vi "GDX-ACC_PitchAndRoll.vi"() -> ()   [LabVIEW 2019]
uses:
  <vilib>/picture/3D Picture Control/Object/Create Object (drawable).vi
  <vilib>/picture/3D Picture Control/NI_3D Picture Control.lvlib
panel:
  in  "Gyro Percent of Filter":dbl(slide)=75.0 scale=0.0..100.0
  out "Filter":refnum<vi>(3d-picture)
  out "Gyro":refnum<vi>(3d-picture)
  out "Accelerometer":refnum<vi>(3d-picture)
  out "Waveform Chart":cluster{dbl, "Radians Out":dbl, "Filtered":dbl}(graph)
  out "error out":errorcluster
  in  "Stop":bool
  in  "Initialize":bool
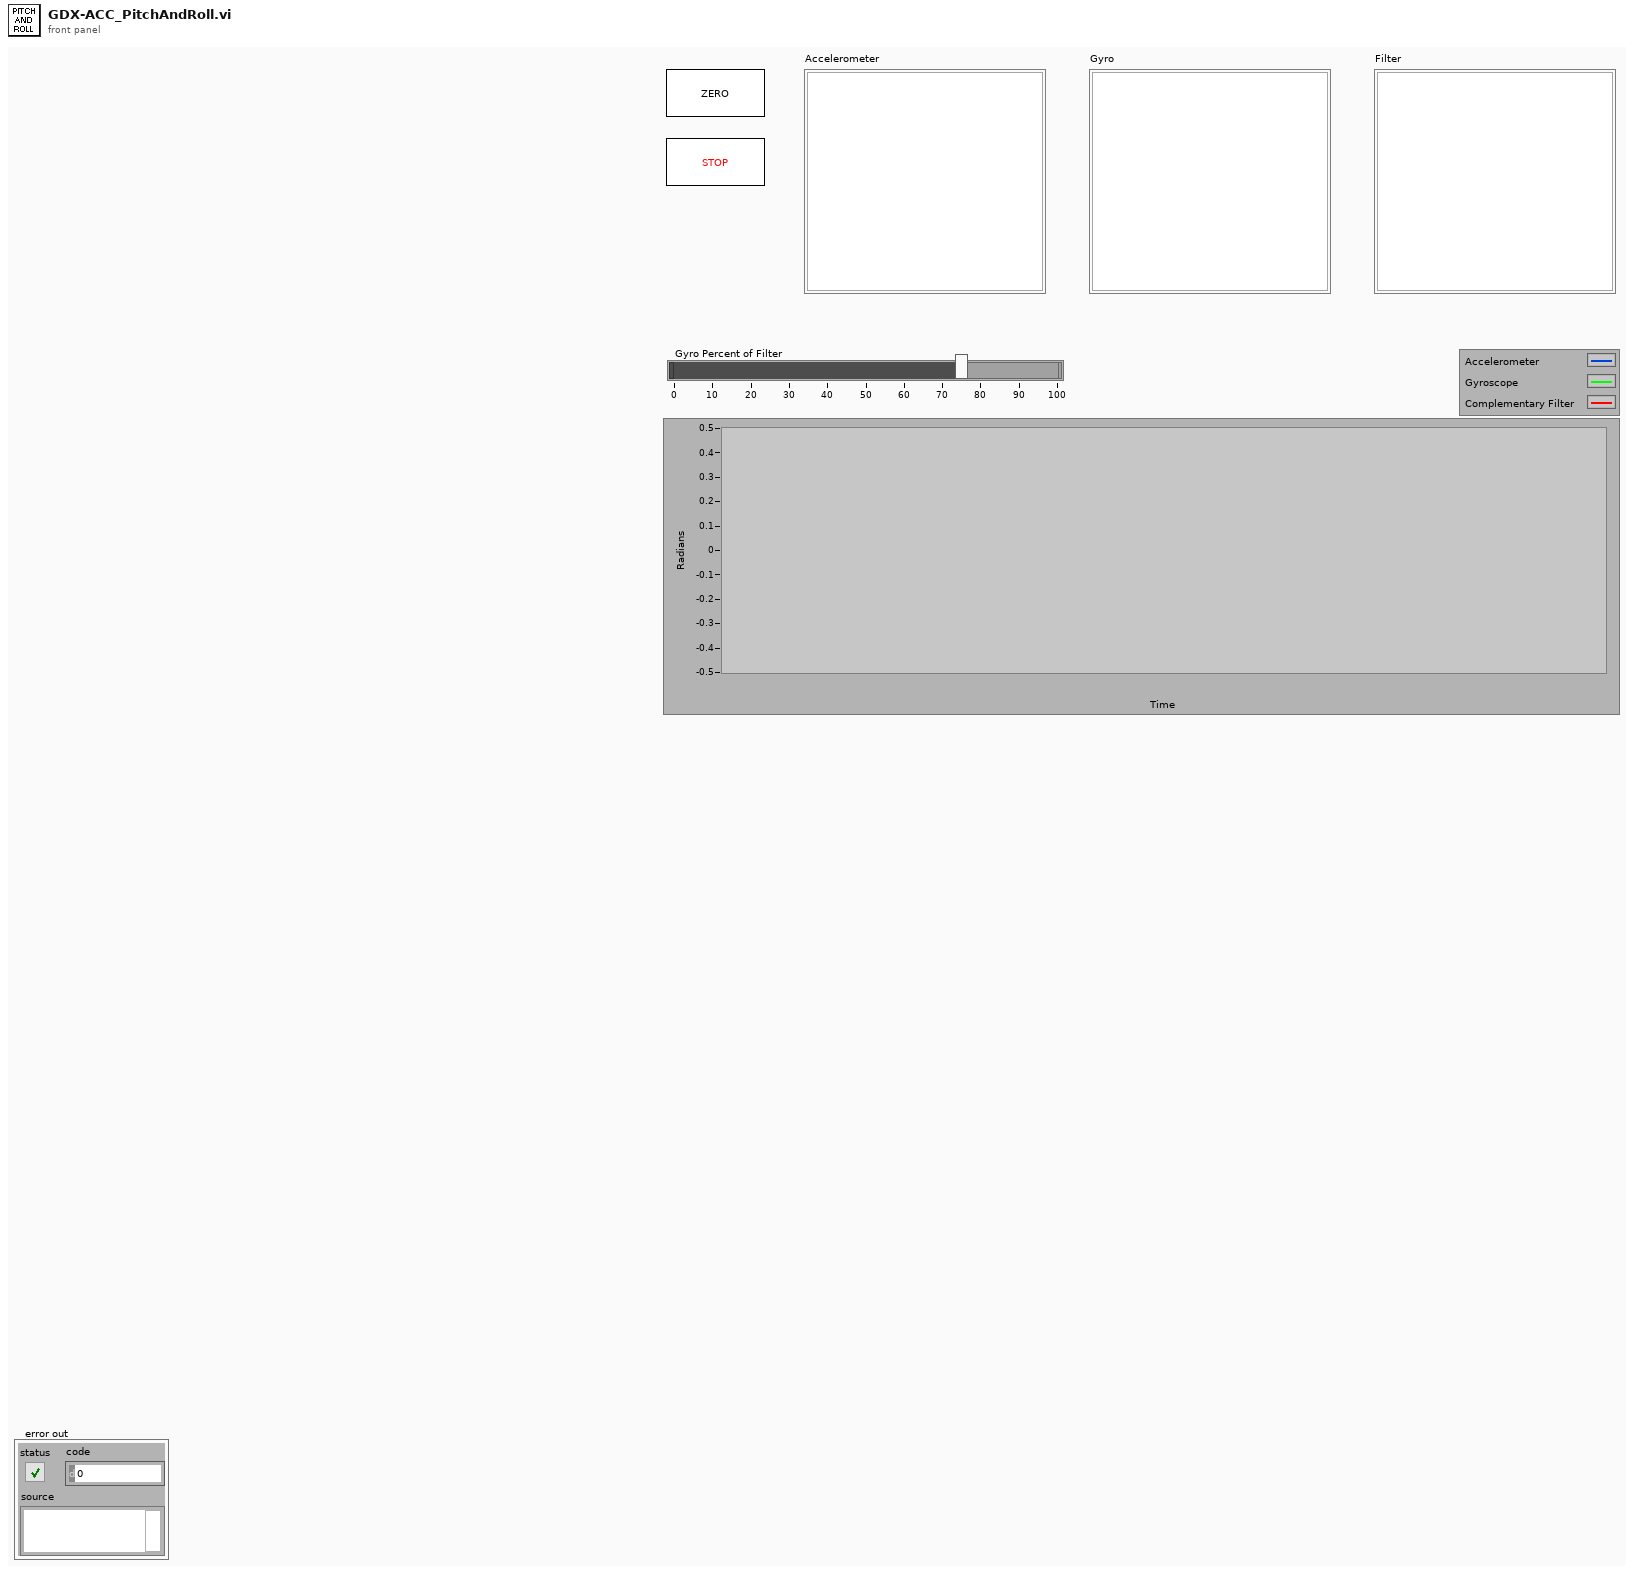
[diagram p1: front panel]
types:
  T1 = enum16{"Activate from Dialog Popup", "Activate All Channels", "Input On/Off Array", "Input Channel  Mask", "Burn Sensor Default Channels"}
  T2 = enum16{"Set Rate from Dialog Popup", "Default 1 Sample/Sec", "Input Sample Rate"}
  T3 = cluster{"Red":sgl, "Green":sgl, "Blue":sgl, "Alpha":sgl}
  T4 = typedef "D2PIO_D2PIOCluster.ctl" = cluster{"Library Handle":i64, "Device List Handle":i64, "BT Device Handles":i64[], "USB Device Handles":i64[], "BT+USB Device Handles":i64[], "Measurement Tick":dbl[], "Ch Availability Mask":u32[]}
  T5 = cluster{"Accel Roll":dbl, "Gyro Roll":dbl, "Filtered Roll":dbl}
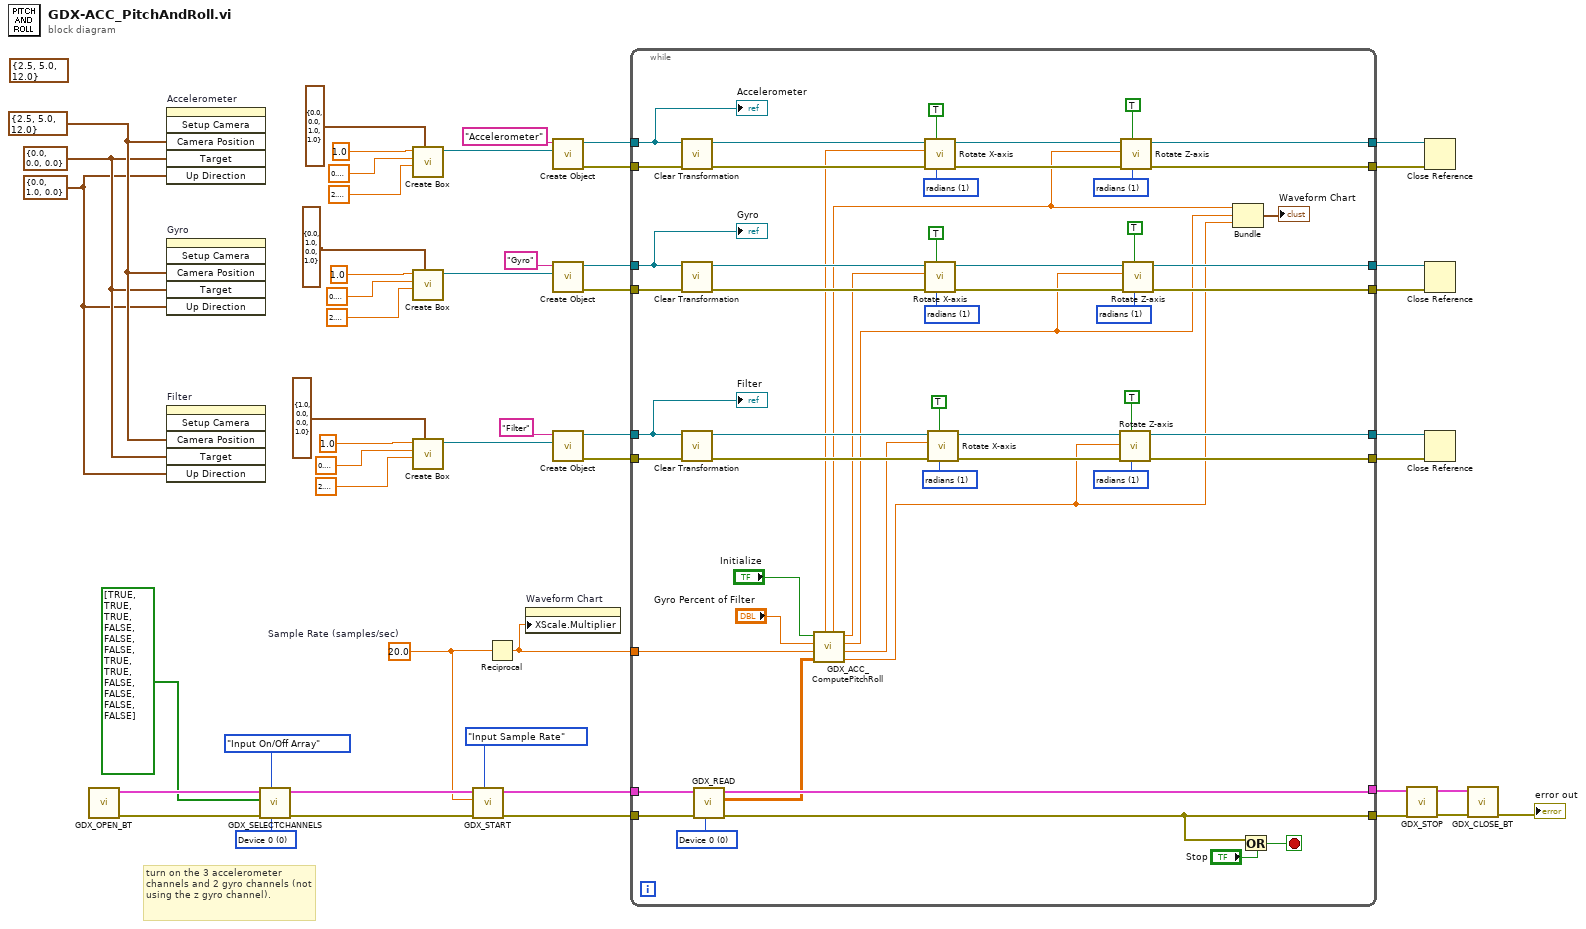
[diagram p0: block diagram]
diagram:
  w4 = 0 items=["Device 0", "Device 1", "Device 2", "Device 3", "Device 4", "Device 5", "Device 6", "Device 7", "Device 8", "Device 9", "Device 10", "Device 11"] ("Device Index")
  w3 = 20.0  # Sample Rate (samples/sec)
  (unwired) cluster{"X":sgl, "Y":sgl, "Z":sgl} {"X"=2.5, "Y"=5.0, "Z"=12.0} ("Camera Position")
  w6 = cluster{"X":sgl, "Y":sgl, "Z":sgl} {"X"=0.0, "Y"=1.0, "Z"=0.0} ("Up Direction")
  w7 = cluster{"X":sgl, "Y":sgl, "Z":sgl} {"X"=0.0, "Y"=0.0, "Z"=0.0} ("Target")
  w8 = cluster{"X":sgl, "Y":sgl, "Z":sgl} {"X"=2.5, "Y"=5.0, "Z"=12.0} ("Camera Position")
  # "turn on the 3 accelerometer channels and 2 gyro channels (not using the z gyro channel)."
  n1 = call <vilib>:"GDX_OPEN_BT.vi"() -> ("error out"=w46:errorcluster, "D2PIO Cluster Out"=w47:T4)  [unwired: 10 in]
  n2 = invoke on="Accelerometer" class="SceneGraphDisp (strict)" method="Setup Camera"("Camera Position"=w8, "Target"=w7, "Up Direction"=w6) -> ()  [unwired: 3 in, 6 out]
  n3 = invoke on="Gyro" class="SceneGraphDisp (strict)" method="Setup Camera"("Camera Position"=w8, "Target"=w7, "Up Direction"=w6) -> ()  [unwired: 3 in, 6 out]
  n4 = invoke on="Filter" class="SceneGraphDisp (strict)" method="Setup Camera"("Camera Position"=w8, "Target"=w7, "Up Direction"=w6) -> ()  [unwired: 3 in, 6 out]
  n5 = call <vilib>:"GDX_SELECTCHANNELS.vi"("Device Index"=w4, "Enum"=T1."Input On/Off Array", "error in (no error)"=w46, "Channel On/Off Array"=bool[] [TRUE, TRUE, TRUE, FALSE, FALSE, FALSE, TRUE, TRUE, FALSE, FALSE, FALSE, FALSE] ("Active Ch Array"), "D2PIO Cluster In"=w47) -> ("error out"=w44:errorcluster, "D2PIO Cluster Out"=w45:T4)  [unwired: 5 in]
  n6 = call <vilib>:"Create Box.vi"("Color"=T3 {"Red"=0.0, "Green"=0.0, "Blue"=1.0, "Alpha"=1.0}, "Length Z"=sgl 2.4, "Length Y"=sgl 0.6, "Length X"=sgl 1.0) -> ("New Box Refnum"=w37:refnum<vi>)  [unwired: 6 in, 1 out]
  n7 = call <vilib>:"Create Box.vi"("Color"=T3 {"Red"=0.0, "Green"=1.0, "Blue"=0.0, "Alpha"=1.0}, "Length Z"=sgl 2.4, "Length Y"=sgl 0.6, "Length X"=sgl 1.0) -> ("New Box Refnum"=w21:refnum<vi>)  [unwired: 6 in, 1 out]
  n8 = call <vilib>:"Create Box.vi"("Color"=T3 {"Red"=1.0, "Green"=0.0, "Blue"=0.0, "Alpha"=1.0}, "Length Z"=sgl 2.4, "Length Y"=sgl 0.6, "Length X"=sgl 1.0) -> ("New Box Refnum"=w18:refnum<vi>)  [unwired: 6 in, 1 out]
  n9 = call <vilib>:"GDX_START.vi"("Enum"=T2."Input Sample Rate", "error in (no error)"=w44, "Sample Rate (samples/sec)"=w3, "D2PIO Cluster In"=w45) -> ("error out"=w43:errorcluster, "D2PIO Cluster Out"=w42:T4)  [unwired: 4 in, 2 out]
  n10 = Reciprocal(x=w3) -> (1/x=w39:dbl)
  n11 = property on="Waveform Chart" class="WFChart (strict)"("XScale.Multiplier"=w39) -> ()  [unwired: 2 in, 2 out]
  n12 = call-poly <vilib>:"Create Object.vi"("Geometry"=w37, "Name"="Accelerometer") -> ("error out"=w35:errorcluster, "Scene:New Object"=w36:refnum<vi>)  [unwired: 8 in]
  n13 = call-poly <vilib>:"Create Object.vi"("Geometry"=w21, "Name"="Gyro") -> ("error out"=w23:errorcluster, "Scene:New Object"=w22:refnum<vi>)  [unwired: 8 in]
  n14 = call-poly <vilib>:"Create Object.vi"("Geometry"=w18, "Name"="Filter") -> ("error out"=w16:errorcluster, "Scene:New Object"=w17:refnum<vi>)  [unwired: 8 in]
  n15 = while {
    tunnel: w43 -> [w100]
    tunnel: w42 -> [w102]
    tunnel: [w101] -> w41
    tunnel: [w99] -> w40
    tunnel: w39 -> [w58]
    tunnel: w36 -> [w94]
    tunnel: w35 -> [w96]
    tunnel: [w92] -> w34
    tunnel: [w90] -> w33
    tunnel: w22 -> [w77]
    tunnel: w23 -> [w75]
    tunnel: [w79] -> w24
    tunnel: [w81] -> w25
    tunnel: w17 -> [w70]
    tunnel: w16 -> [w72]
    tunnel: [w68] -> w15
    tunnel: [w66] -> w14
    stop <- w104 stop-if-true
    w63 = u16 1 items=["degree", "radians"] ("angle unit")
    w65 = u16 1 items=["degree", "radians"] ("angle unit")
    w84 = u16 1 items=["degree", "radians"] ("angle unit")
    w82 = u16 1 items=["degree", "radians"] ("angle unit")
    w87 = u16 1 items=["degree", "radians"] ("angle unit")
    w89 = u16 1 items=["degree", "radians"] ("angle unit")
    w98 = 0 items=["Device 0", "Device 1", "Device 2", "Device 3", "Device 4", "Device 5", "Device 6", "Device 7", "Device 8", "Device 9", "Device 10", "Device 11"] ("Device Index")
    n16 = call <vilib>:"Clear Transformation.vi"("error in (no error)"=w96, "Object Refnum In"=w94) -> ("error out"=w97:errorcluster, "Object Refnum Out"=w95:refnum<vi>)  [unwired: 8 out]
    n17 = call <vilib>:"Clear Transformation.vi"("error in (no error)"=w75, "Object Refnum In"=w77) -> ("error out"=w74:errorcluster, "Object Refnum Out"=w76:refnum<vi>)  [unwired: 8 out]
    n18 = call <vilib>:"Clear Transformation.vi"("error in (no error)"=w72, "Object Refnum In"=w70) -> ("error out"=w73:errorcluster, "Object Refnum Out"=w71:refnum<vi>)  [unwired: 8 out]
    n19 = call <vilib>:"GDX_READ.vi"("Device Index"=w98, "error in (no error)"=w100, "D2PIO Cluster In"=w102) -> ("error out"=w99:errorcluster, "Waveform Chart Data"=w59:dbl[][], "D2PIO Cluster Out"=w101:T4)  [unwired: 3 in, 3 out]
    n20 = call "GDX_ACC_ComputePitchRoll.vi"("Measurements In"=w59, "dt"=w58, "Gyro Percent of Filter"="Gyro Percent of Filter", "Initialize"="Initialize") -> ("Filtered Roll"=w51:dbl, "Filtered Pitch"=w54:dbl, "Gyro Roll"=w52:dbl, "Gyro Pitch"=w55:dbl, "Accel Roll"=w56:dbl, "Accel Pitch"=w57:dbl)  [unwired: 2 in]
    n21 = call <vilib>:"Rotate X-axis.vi"("angle unit"=w89, "Relative?"=TRUE, "error in (no error)"=w97, "angle"=w57, "Scene Object In"=w95) -> ("error out"=w91:errorcluster, "Scene Object Out"=w93:refnum<vi>)  [unwired: 5 in]
    n22 = call <vilib>:"Rotate X-axis.vi"("angle unit"=w82, "Relative?"=TRUE, "error in (no error)"=w74, "angle"=w55, "Scene Object In"=w76) -> ("error out"=w80:errorcluster, "Scene Object Out"=w78:refnum<vi>)  [unwired: 5 in]
    n23 = call <vilib>:"Rotate X-axis.vi"("angle unit"=w65, "Relative?"=TRUE, "error in (no error)"=w73, "angle"=w54, "Scene Object In"=w71) -> ("error out"=w67:errorcluster, "Scene Object Out"=w69:refnum<vi>)  [unwired: 5 in]
    n24 = call <vilib>:"Rotate Z-axis.vi"("angle unit"=w63, "Relative?"=TRUE, "error in (no error)"=w67, "angle"=w51, "Scene Object In"=w69) -> ("error out"=w66:errorcluster, "Scene Object Out"=w68:refnum<vi>)  [unwired: 5 in]
    n25 = call <vilib>:"Rotate Z-axis.vi"("angle unit"=w87, "Relative?"=TRUE, "error in (no error)"=w91, "angle"=w56, "Scene Object In"=w93) -> ("error out"=w90:errorcluster, "Scene Object Out"=w92:refnum<vi>)  [unwired: 5 in]
    n26 = call <vilib>:"Rotate Z-axis.vi"("angle unit"=w84, "Relative?"=TRUE, "error in (no error)"=w80, "angle"=w52, "Scene Object In"=w78) -> ("error out"=w81:errorcluster, "Scene Object Out"=w79:refnum<vi>)  [unwired: 5 in]
    n27 = Bundle("Accel Roll"=w56, "Gyro Roll"=w52, "Filtered Roll"=w51) -> (→"Waveform Chart":T5)  [unwired: 1 in]
    n28 = Or(x=w99, y="Stop") -> (x .or. y?=w104:bool)
    "Accelerometer" <- w94
    "Gyro" <- w77
    "Filter" <- w70
  }
  n29 = call <vilib>:"GDX_STOP.vi"("error in (no error)"=w40, "D2PIO Cluster In"=w41) -> ("error out"=w49:errorcluster, "D2PIO Cluster Out"=w50:T4)  [unwired: 8 in]
  n30 = Close Reference(reference=w34, error in (no error)=w33) -> ()  [unwired: 1 out]
  n31 = Close Reference(reference=w24, error in (no error)=w25) -> ()  [unwired: 1 out]
  n32 = Close Reference(reference=w15, error in (no error)=w14) -> ()  [unwired: 1 out]
  n33 = call <vilib>:"GDX_CLOSE_BT.vi"("error in (no error)"=w49, "D2PIO Cluster In"=w50) -> ("error out"=→"error out":errorcluster)  [unwired: 8 in, 1 out]
